vi "String Escape.vi"(11 "Unescaped String":string) -> (3 "Escaped String":string)   [LabVIEW 2017, in "LabVIEW-Config.lvlib" / "LabVIEW-Config.lvclass"]
uses:
  LabVIEW-Config.lvclass
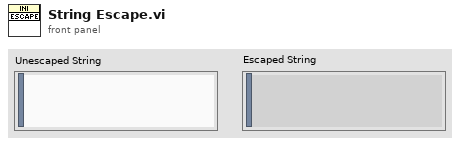
[diagram p1: front panel]
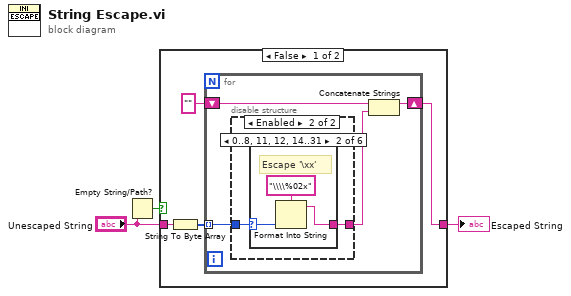
[diagram p0: block diagram]
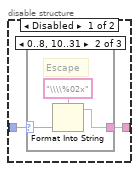
[diagram p2: hidden frame]
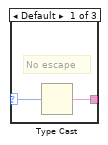
[diagram p3: hidden frame]
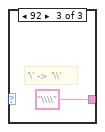
[diagram p4: hidden frame]
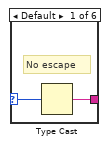
[diagram p5: hidden frame]
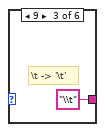
[diagram p6: hidden frame]
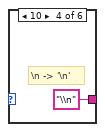
[diagram p7: hidden frame]
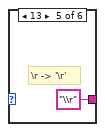
[diagram p8: hidden frame]
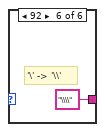
[diagram p9: hidden frame]
diagram:
  n1 = Empty String/Path?(string/path="Unescaped String") -> (empty?=w1:bool)
  n2 = case shown="False" w1 {
    tunnel: "Unescaped String" -> [w6 w31]
    tunnel: [w4 w31] -> w3
    frame False {
      n3 = String To Byte Array(string=w6) -> (unsigned byte array=w7:u8[])
      n4 = for {
        tunnel: w7 -> [w11] mode=indexing
        shift-right: [w9] -> w4
        shift-left: "" -> [w10]
        n5 = disable-structure shown="Enabled" {
          disable-tunnel: w11 -> [w13 w21]
          disable-tunnel: [w12 w20] -> w8
          frame Disabled {
            n6 = case shown="0..8, 10..31" w13 {
              selector: w13 -> [w15 w17 _]
              tunnel: [w14 w16 "\\\\" ("Format String")] -> w12
              frame Default {
                # "No escape"
                n7 = Type Cast(x=w15) -> (*(type *) &x=w14:string)  [unwired: 1 in]
              }
              frame 0..8, 10..31 {
                # "Escape"
                n8 = Format Into String(format string="\\\\%02x" ("Format String"), w17) -> (resulting string=w16:string)  [unwired: 2 in, 1 out]
              }
              frame 92 {
                # "'\\' -> '\\\\'"
              }
            }
          }
          frame Enabled {
            n9 = case shown="0..8, 11, 12, 14..31" w21 {
              selector: w21 -> [w23 w25 _ _ _ _]
              tunnel: [w22 w24 "\\t" ("Format String") "\\n" ("Format String") "\\r" ("Format String") "\\\\" ("Format String")] -> w20
              frame Default {
                # "No escape"
                n10 = Type Cast(x=w23) -> (*(type *) &x=w22:string)  [unwired: 1 in]
              }
              frame 0..8, 11, 12, 14..31 {
                # "Escape '\\xx'"
                n11 = Format Into String(format string="\\\\%02x" ("Format String"), w25) -> (resulting string=w24:string)  [unwired: 2 in, 1 out]
              }
              frame 9 {
                # "\\t -> '\\t'"
              }
              frame 10 {
                # "\\n -> '\\n'"
              }
              frame 13 {
                # "\\r -> '\\r'"
              }
              frame 92 {
                # "'\\' -> '\\\\'"
              }
            }
          }
        }
        n12 = Concatenate Strings(w10, w8) -> (w9:string)
      }
    }
    frame True {
    }
  }
  "Escaped String" <- w3
